vi "ZCAN_ReceiveByType.vi"(8 "error in (no error)":errorcluster, 9 "Agreement":u32, 11 "Can_CH_handle":u32) -> (0 "error out":errorcluster, 1 "Receive_Num":u32, 3 "CAN DATA":string)   [LabVIEW 2020, in "zlgcan.lvlib"]
uses:
  zlgcan.lvlib
  bin/zlgcan_wrap.dll
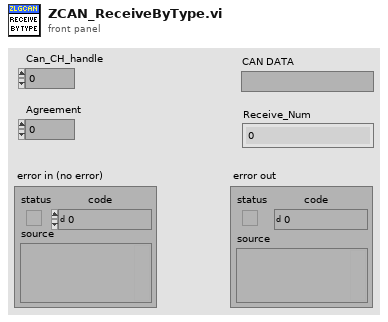
[diagram p1: front panel]
types:
  T1 = cluster{"[0]":u8, "[1]":u8, "[2]":u8, "[3]":u8, "[4]":u8, "[5]":u8, "[6]":u8, "[7]":u8, "[8]":u8, "[9]":u8, "[10]":u8, "[11]":u8, "[12]":u8, "[13]":u8, "[14]":u8, "[15]":u8, "[16]":u8, "[17]":u8, "[18]":u8, "[19]":u8, "[20]":u8, "[21]":u8, "[22]":u8, "[23]":u8, "[24]":u8, "[25]":u8, "[26]":u8, "[27]":u8, "[28]":u8, "[29]":u8, "[30]":u8, "[31]":u8, "[32]":u8, "[33]":u8, "[34]":u8, "[35]":u8, "[36]":u8, "[37]":u8, "[38]":u8, "[39]":u8, "[40]":u8, "[41]":u8, "[42]":u8, "[43]":u8, "[44]":u8, "[45]":u8, "[46]":u8, "[47]":u8, "[48]":u8, "[49]":u8, "[50]":u8, "[51]":u8, "[52]":u8, "[53]":u8, "[54]":u8, "[55]":u8, "[56]":u8, "[57]":u8, "[58]":u8, "[59]":u8, "[60]":u8, "[61]":u8, "[62]":u8, "[63]":u8}
  T2 = cluster{u32, u8, u8, u8, u8, cluster{"[0]":u8, "[1]":u8, "[2]":u8, "[3]":u8, "[4]":u8, "[5]":u8, "[6]":u8, "[7]":u8, "[8]":u8, "[9]":u8, "[10]":u8, "[11]":u8, "[12]":u8, "[13]":u8, "[14]":u8, "[15]":u8, "[16]":u8, "[17]":u8, "[18]":u8, "[19]":u8, "[20]":u8, "[21]":u8, "[22]":u8, "[23]":u8, "[24]":u8, "[25]":u8, "[26]":u8, "[27]":u8, "[28]":u8, "[29]":u8, "[30]":u8, "[31]":u8, "[32]":u8, "[33]":u8, "[34]":u8, "[35]":u8, "[36]":u8, "[37]":u8, "[38]":u8, "[39]":u8, "[40]":u8, "[41]":u8, "[42]":u8, "[43]":u8, "[44]":u8, "[45]":u8, "[46]":u8, "[47]":u8, "[48]":u8, "[49]":u8, "[50]":u8, "[51]":u8, "[52]":u8, "[53]":u8, "[54]":u8, "[55]":u8, "[56]":u8, "[57]":u8, "[58]":u8, "[59]":u8, "[60]":u8, "[61]":u8, "[62]":u8, "[63]":u8}, u64}
  T3 = cluster{u32, u8, u8, u8, u8, cluster{"[0]":u8, "[1]":u8, "[2]":u8, "[3]":u8, "[4]":u8, "[5]":u8, "[6]":u8, "[7]":u8, "[8]":u8, "[9]":u8, "[10]":u8, "[11]":u8, "[12]":u8, "[13]":u8, "[14]":u8, "[15]":u8, "[16]":u8, "[17]":u8, "[18]":u8, "[19]":u8, "[20]":u8, "[21]":u8, "[22]":u8, "[23]":u8, "[24]":u8, "[25]":u8, "[26]":u8, "[27]":u8, "[28]":u8, "[29]":u8, "[30]":u8, "[31]":u8, "[32]":u8, "[33]":u8, "[34]":u8, "[35]":u8, "[36]":u8, "[37]":u8, "[38]":u8, "[39]":u8, "[40]":u8, "[41]":u8, "[42]":u8, "[43]":u8, "[44]":u8, "[45]":u8, "[46]":u8, "[47]":u8, "[48]":u8, "[49]":u8, "[50]":u8, "[51]":u8, "[52]":u8, "[53]":u8, "[54]":u8, "[55]":u8, "[56]":u8, "[57]":u8, "[58]":u8, "[59]":u8, "[60]":u8, "[61]":u8, "[62]":u8, "[63]":u8}, u64}[]
  T4 = cluster{"[0]":u8, "[1]":u8, "[2]":u8, "[3]":u8, "[4]":u8, "[5]":u8, "[6]":u8, "[7]":u8}
  T5 = cluster{u32, u8, u8, u8, u8, cluster{"[0]":u8, "[1]":u8, "[2]":u8, "[3]":u8, "[4]":u8, "[5]":u8, "[6]":u8, "[7]":u8}, u64}
  T6 = cluster{u32, u8, u8, u8, u8, cluster{"[0]":u8, "[1]":u8, "[2]":u8, "[3]":u8, "[4]":u8, "[5]":u8, "[6]":u8, "[7]":u8}, u64}[]
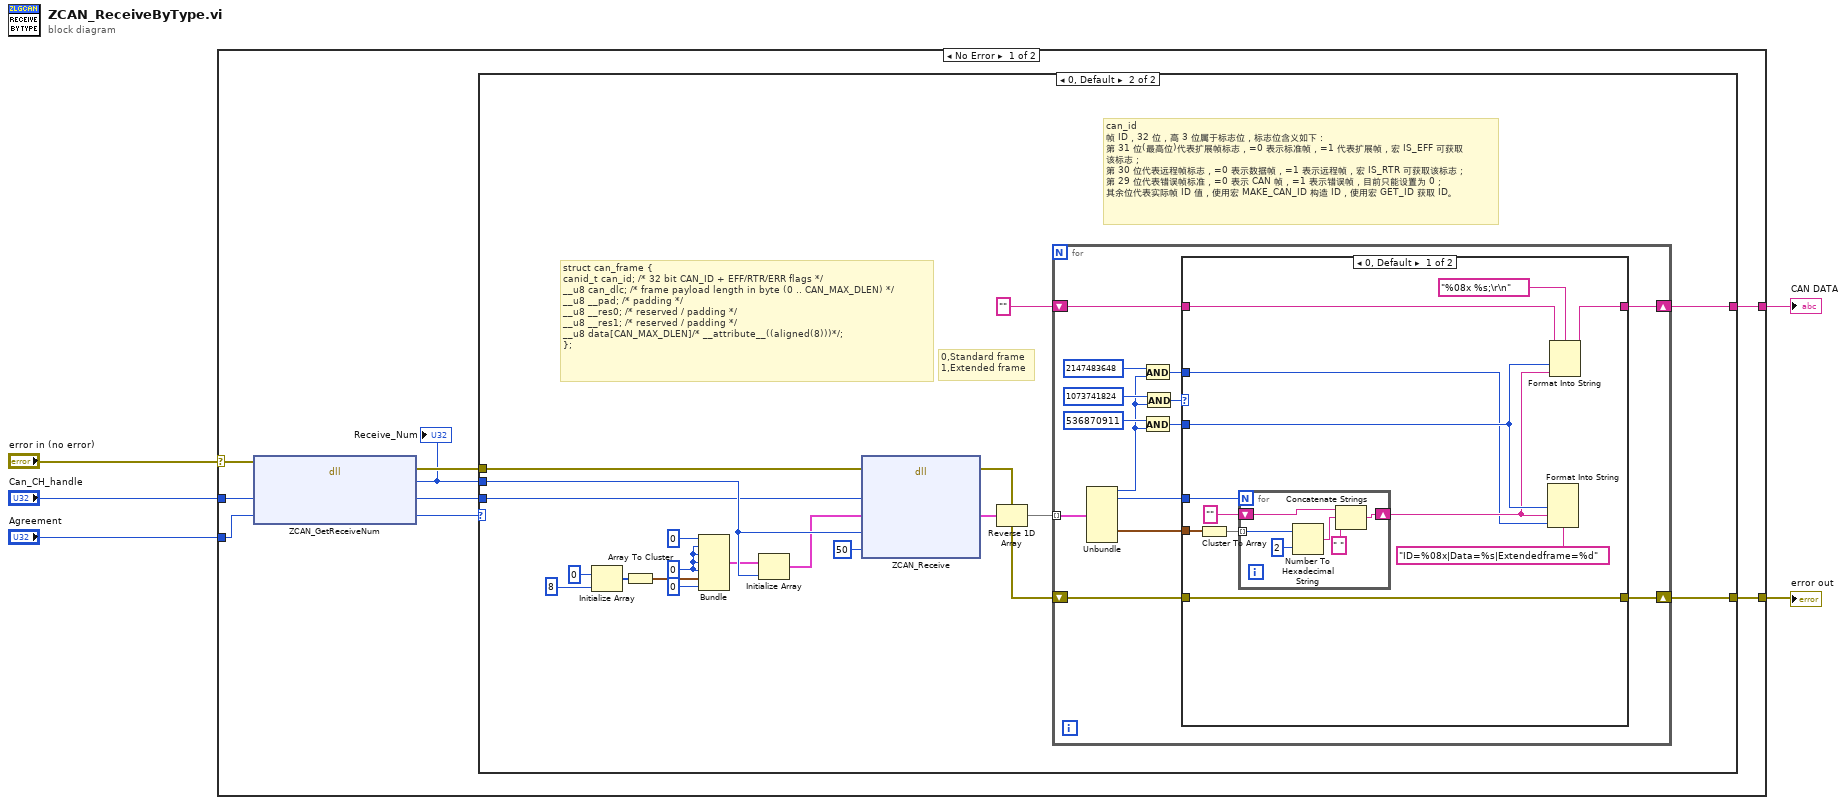
[diagram p0: block diagram]
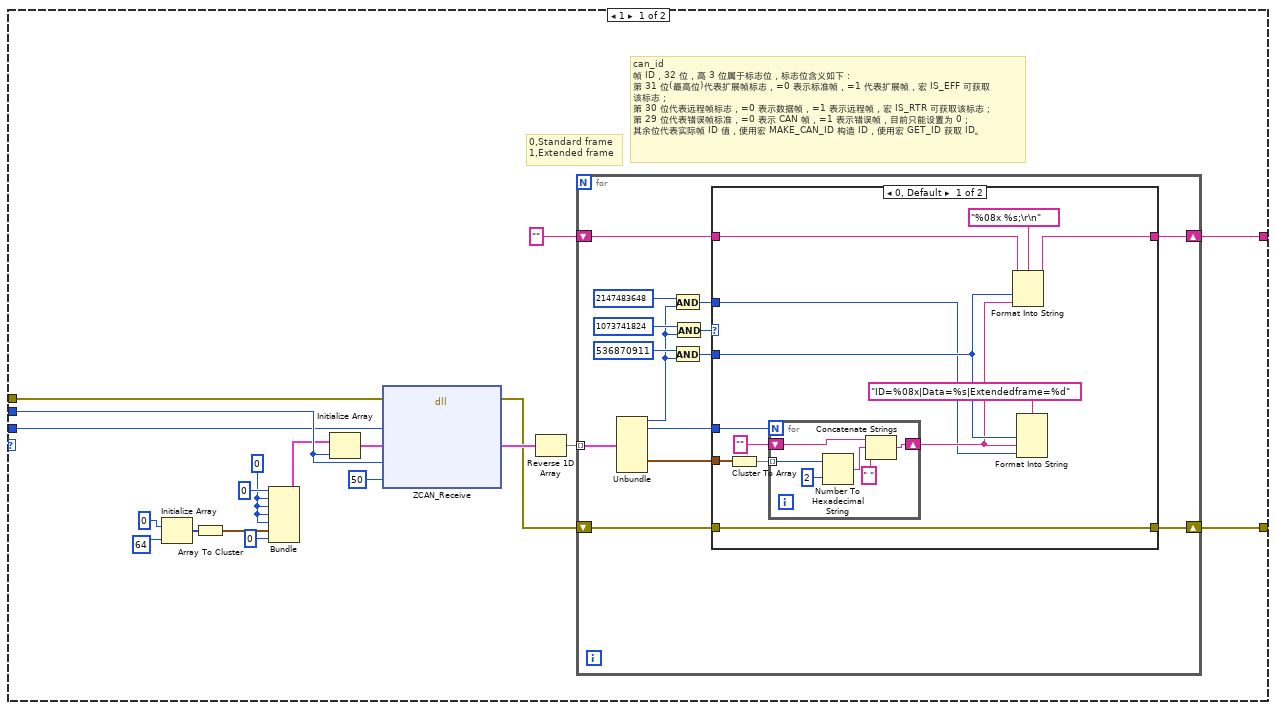
[diagram p2: hidden frame]
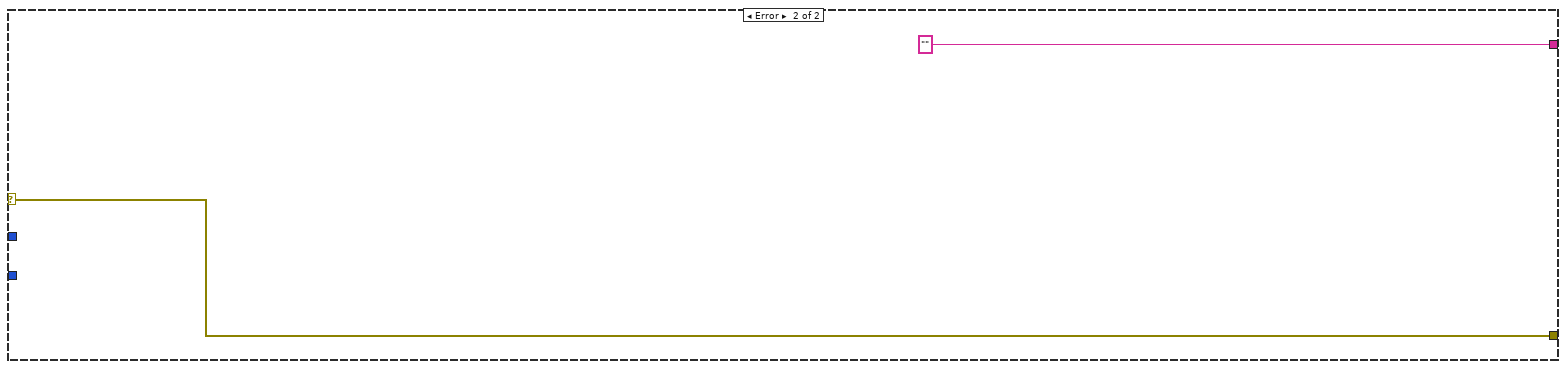
[diagram p5: hidden frame]
diagram:
  n1 = case shown="No Error" "error in (no error)" {
    selector: "error in (no error)" -> [w10 w122]
    tunnel: "Can_CH_handle" -> [w14 _]
    tunnel: "Agreement" -> [w13 _]
    tunnel: [w11 ""] -> w3
    tunnel: [w8 w122] -> w1
    frame No Error {
      n2 = dll-call lib="D:/Git/ZLG_USBCANFD/bin/zlgcan_wrap.dll" fn="ZCAN_GetReceiveNum"(error in=w10, "通道句柄"=w14, "协议"=w13) -> (error out=w12:errorcluster, "缓冲区帧数"=w6:u32, "通道句柄"=w9:u32, "协议"=w7:u8)  [unwired: 2 in, 1 out]
      "Receive_Num" <- w6
      n3 = case shown="0, Default" w7 {
        tunnel: w6 -> [w32 w85]
        tunnel: w12 -> [w33 w86]
        tunnel: [w30 w84] -> w11
        tunnel: w9 -> [w29 w83]
        tunnel: [w27 w81] -> w8
        frame 1 {
          w20 = u8 0
          # "0,Standard frame\n1,Extended frame"
          # "can_id\n帧 ID，32 位，高 3 位属于标志位，标志位含义如下：\n第 31 位(最高位)代表扩展帧标志，=0 表示标准帧，=1 代表扩展帧，宏 IS_EFF 可获取\n该标志；\n第 30 位代表远程帧标志，=0 表示数据帧，=1 表示远程帧，宏 IS_RTR 可获取该标志；\n第 29 位代表错误帧标准，=0 表示 CAN 帧，=1 表示错误帧，目前只能设置为 0；\n其余位代表实际帧 ID 值，使用宏 MAKE_CAN_ID 构造 ID，使用宏 GET_ID 获取 ID。"
          n4 = Initialize Array(u8 0 ("元素"), u32 64 ("维数大小")) -> (w22:u8[])
          n5 = Array To Cluster(array=w22) -> (cluster=w23:T1)
          n6 = Bundle(u32 0, w20, w20, w20, w20, w23, u64 0) -> (w24:T2)  [unwired: 1 in]
          n7 = Initialize Array(w24, w32) -> (w16:T3)
          n8 = dll-call lib="D:/Git/ZLG_USBCANFD/bin/zlgcan_wrap.dll" fn="ZCAN_Receive"(error in=w33, "通道句柄"=w29, "数据帧数组"=w16, "数据帧数"=w32, "超时时间"=50) -> (error out=w28:errorcluster, "数据帧数组"=w31:T3)  [unwired: 6 in, 1 out]
          n9 = Reverse 1D Array(array=w31) -> (reversed array=w25:T3)
          n10 = for {
            tunnel: w25 -> [w47] mode=indexing
            shift-right: [w37] -> w30
            shift-left: "" -> [w36]
            shift-right: [w34] -> w27
            shift-left: w28 -> [w35]
            n11 = Unbundle(w47) -> (w43:u32, w40:u8, w39:T1)  [unwired: 4 out]
            n12 = And(x=u32 2147483648, y=w43) -> (x .and. y?=w38:u32)
            n13 = And(x=u32 536870911, y=w43) -> (x .and. y?=w41:u32)
            n14 = And(x=u32 1073741824, y=w43) -> (x .and. y?=w42:u32)
            n15 = case shown="0, Default" w42 {
              tunnel: w41 -> [w52 _]
              tunnel: w40 -> [w56 _]
              tunnel: w39 -> [w59 _]
              tunnel: w38 -> [w50 _]
              tunnel: [w55 w67] -> w37
              tunnel: w36 -> [w54 w67]
              tunnel: w35 -> [w48 w66]
              tunnel: [w48 w66] -> w34
              frame 0, Default {
                n16 = Cluster To Array(cluster=w59) -> (array=w58:u8[])
                n17 = for {
                  N: w56 -> [_]
                  shift-right: [w62] -> w51
                  shift-left: "" -> [w60]
                  tunnel: w58 -> [w61] mode=indexing
                  n18 = Number To Hexadecimal String(1:i16 2 ("width (-)"), 2:w61) -> (0:w64:string)
                  n19 = Concatenate Strings(w60, w64, " " ("string")) -> (w62:string)
                }
                n20 = Format Into String(format string="%08x %s;\r\n", initial string=w54, w52, w51) -> (resulting string=w55:string)  [unwired: 1 in, 1 out]
                n21 = Format Into String(format string="ID=%08x|Data=%s|Extendedframe=%d", w52, w51, w50) -> ()  [unwired: 2 in, 2 out]
              }
              frame 1 {
              }
            }
          }
        }
        frame 0, Default {
          w74 = u8 0
          # "struct can_frame {\ncanid_t can_id; /* 32 bit CAN_ID + EFF/RTR/ERR flags */\n__u8 can_dlc; /* frame payload length in byte (0 .. CAN_MAX_DLEN) */\n__u8 __pad; /* padding */\n__u8 __res0; /* reserved / padding */\n__u8 __res1; /* reserved / padding */\n__u8 data[CAN_MAX_DLEN]/* __attribute__((aligned(8)))*/;\n};"
          # "0,Standard frame\n1,Extended frame"
          # "can_id\n帧 ID，32 位，高 3 位属于标志位，标志位含义如下：\n第 31 位(最高位)代表扩展帧标志，=0 表示标准帧，=1 代表扩展帧，宏 IS_EFF 可获取\n该标志；\n第 30 位代表远程帧标志，=0 表示数据帧，=1 表示远程帧，宏 IS_RTR 可获取该标志；\n第 29 位代表错误帧标准，=0 表示 CAN 帧，=1 表示错误帧，目前只能设置为 0；\n其余位代表实际帧 ID 值，使用宏 MAKE_CAN_ID 构造 ID，使用宏 GET_ID 获取 ID。"
          n22 = Initialize Array(u8 0 ("元素"), u32 8 ("维数大小")) -> (w76:u8[])
          n23 = Array To Cluster(array=w76) -> (cluster=w77:T4)
          n24 = Bundle(u32 0, w74, w74, w74, w74, w77, u64 0) -> (w78:T5)  [unwired: 1 in]
          n25 = Initialize Array(w78, w85) -> (w70:T6)
          n26 = dll-call lib="D:/Git/ZLG_USBCANFD/bin/zlgcan_wrap.dll" fn="ZCAN_Receive"(error in=w86, "通道句柄"=w83, "数据帧数组"=w70, "数据帧数"=w85, "超时时间"=50) -> (error out=w82:errorcluster, "数据帧数组"=w68:T6)  [unwired: 6 in, 1 out]
          n27 = Reverse 1D Array(array=w68) -> (reversed array=w79:T6)
          n28 = for {
            tunnel: w79 -> [w100] mode=indexing
            shift-right: [w90] -> w84
            shift-left: "" -> [w89]
            shift-right: [w87] -> w81
            shift-left: w82 -> [w88]
            n29 = Unbundle(w100) -> (w96:u32, w93:u8, w92:T4)  [unwired: 4 out]
            n30 = And(x=u32 2147483648, y=w96) -> (x .and. y?=w91:u32)
            n31 = And(x=u32 536870911, y=w96) -> (x .and. y?=w94:u32)
            n32 = And(x=u32 1073741824, y=w96) -> (x .and. y?=w95:u32)
            n33 = case shown="0, Default" w95 {
              tunnel: w94 -> [w105 _]
              tunnel: w93 -> [w109 _]
              tunnel: w92 -> [w112 _]
              tunnel: w91 -> [w103 _]
              tunnel: [w108 w120] -> w90
              tunnel: w89 -> [w107 w120]
              tunnel: w88 -> [w101 w119]
              tunnel: [w101 w119] -> w87
              frame 0, Default {
                n34 = Cluster To Array(cluster=w112) -> (array=w111:u8[])
                n35 = for {
                  N: w109 -> [_]
                  shift-right: [w115] -> w104
                  shift-left: "" -> [w113]
                  tunnel: w111 -> [w114] mode=indexing
                  n36 = Number To Hexadecimal String(1:i16 2 ("width (-)"), 2:w114) -> (0:w117:string)
                  n37 = Concatenate Strings(w113, w117, " " ("string")) -> (w115:string)
                }
                n38 = Format Into String(format string="ID=%08x|Data=%s|Extendedframe=%d", w105, w104, w103) -> ()  [unwired: 2 in, 2 out]
                n39 = Format Into String(format string="%08x %s;\r\n", initial string=w107, w105, w104) -> (resulting string=w108:string)  [unwired: 1 in, 1 out]
              }
              frame 1 {
              }
            }
          }
        }
      }
    }
    frame Error {
    }
  }
  "CAN DATA" <- w3
  "error out" <- w1
